vi "Measure Waveform.vi"(8 "error in":errorcluster, 9 "timeout[s]":dbl=10.0 format="%0.2f", 10 "number of samples per channel":i32=-1, 11 "task/channels in":string) -> (0 "error out":errorcluster, 2 "data":waveform(dbl)[](array[waveform]), 3 "task out":refnum<k21>)   [LabVIEW 2023, in "AI.lvlib"]
uses:
  AI.lvlib
  <vilib>/DAQmx/read.llb/DAQmx Read (Analog 1D Wfm NChan NSamp).vi
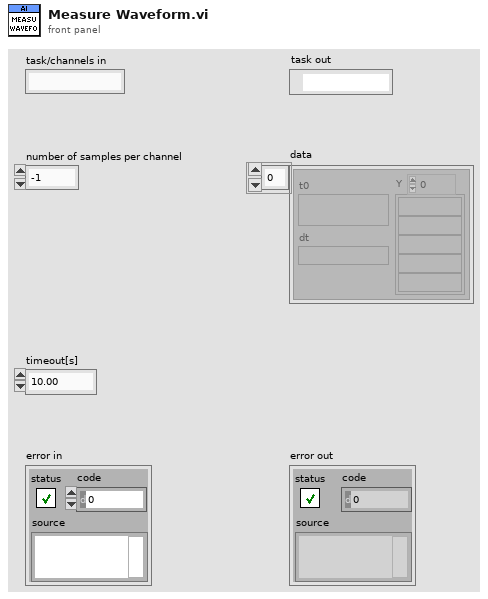
[diagram p1: front panel]
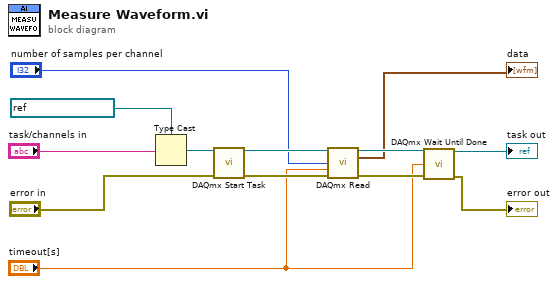
[diagram p0: block diagram]
diagram:
  n1 = Type Cast(type=refnum<k21> "Station2_DUT1" ("task/channels in"), x="task/channels in") -> (*(type *) &x=w1:refnum<k21>)
  n2 = call <vilib>:"DAQmx Start Task.vi"("task/channels in"=w1, "error in"="error in") -> ("task out"=w12:refnum<k21>, "error out"=w11:errorcluster)  [unwired: 12 in]
  n3 = call-poly <vilib>:"DAQmx Read.vi"("task/channels in"=w12, "number of samples per channel"="number of samples per channel", "timeout"="timeout[s]", "error in"=w11) -> ("task out"=w9:refnum<k21>, "data"=→"data":waveform(dbl)[], "error out"=w8:errorcluster)  [unwired: 9 in]
  n4 = call <vilib>:"DAQmx Wait Until Done.vi"("task/channels in"=w9, "timeout (sec)"="timeout[s]", "error in"=w8) -> ("task out"=→"task out":refnum<k21>, "error out"=→"error out":errorcluster)  [unwired: 11 in]
